vi "Draw TextBox.vi"(7 "heading (rad)":dbl, 9 "draw options":T1={"Outer Border Color"=0, "Inner Border Color"=6316128, "Outer Gradient Color"=2565927, "Inner Gradient Color"=16860, "Compass North Pointer Color"=16711680, "Compass Pointer Color 1"=13355429, "Compass Pointer Color 2"=14934973, "Direction Pointer Color"=16765184, "Text Box Outline Color"=13355429, "Text Box Background Color"=14934973, "Scale Color"=16448250, "Text Color"=0, "Draw Gradient"=TRUE, "Draw Rose"=TRUE, "Simple Scale"=TRUE, "Draw Text"=FALSE, "Font Name"="Helvetica", "Angle Units"=enum."Degrees"}, 10 "draw area cache":T3, 11 "picture in":picture) -> (3 "picture out":picture)   [LabVIEW 2017, in "NI_Robotics_Compass Picture.lvlib"]
uses:
  <vilib>/robotics/Controls/Compass Indicator/Compass Picture/NI_Robotics_Compass Picture.lvlib
  <vilib>/robotics/Controls/Compass Indicator/Compass Picture/Draw Area State.ctl
  <vilib>/Utility/miscctls.llb/LVBoundsTypeDef.ctl
  <vilib>/robotics/Controls/Compass Indicator/Compass Picture/Draw Options.ctl
  <vilib>/robotics/Controls/Utilities/Angle Units.ctl
  <vilib>/picture/picture.llb/Get Text Rect.vi
  <vilib>/Utility/AngleManip/Radians to Degrees.vi
  <vilib>/Utility/AngleManip/Radians to Degrees (Scalar DBL).vi
  <vilib>/robotics/Controls/Utilities/NI_Robotics_Control Utilities.lvlib
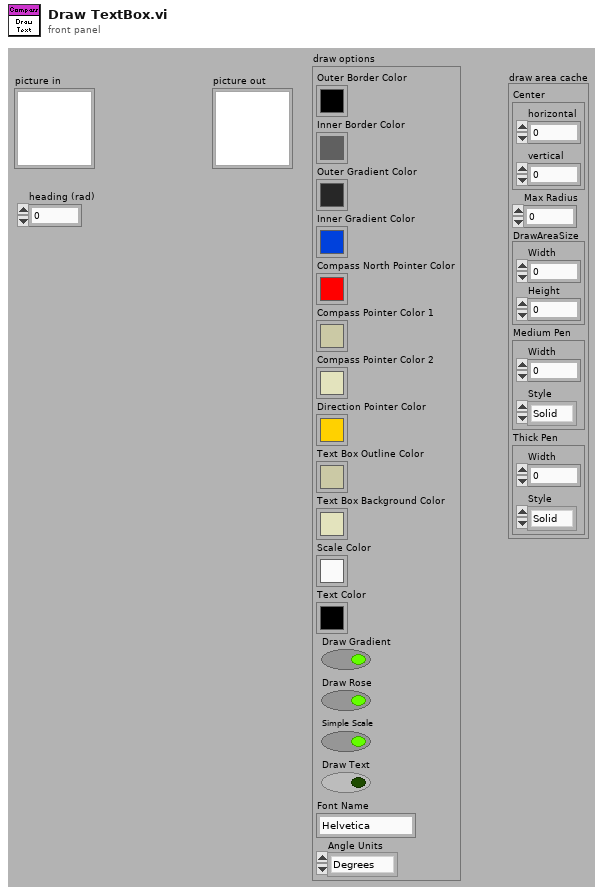
[diagram p1: front panel]
types:
  T1 = typedef "NI_Robotics_Compass Picture.lvlib/Draw Options.ctl" = cluster{"Outer Border Color":u32, "Inner Border Color":u32, "Outer Gradient Color":u32, "Inner Gradient Color":u32, "Compass North Pointer Color":u32, "Compass Pointer Color 1":u32, "Compass Pointer Color 2":u32, "Direction Pointer Color":u32, "Text Box Outline Color":u32, "Text Box Background Color":u32, "Scale Color":u32, "Text Color":u32, "Draw Gradient":bool, "Draw Rose":bool, "Simple Scale":bool, "Draw Text":bool, "Font Name":string, "Angle Units":T2}
  T2 = typedef "NI_Robotics_Control Utilities.lvlib/Angle Units.ctl" = enum16{"Radians", "Degrees"}
  T3 = typedef "NI_Robotics_Compass Picture.lvlib/Draw Area State.ctl" = cluster{"Center":cluster{"horizontal":i16, "vertical":i16}, "Max Radius":dbl, "DrawAreaSize":T4, "Medium Pen":cluster{"Width":u16, "Style":enum32{"Solid", "Dash", "Dot", "DashDot", "DashDotDot"}}, "Thick Pen":cluster{"Width":u16, "Style":enum32{"Solid", "Dash", "Dot", "DashDot", "DashDotDot"}}}
  T4 = typedef "LVBoundsTypeDef.ctl" = cluster{"Width":u32, "Height":u32}
  T5 = cluster{"horizontal":enum16{"left", "center", "right"}, "vertical":enum16{"top", "center", "bottom"}}
  T6 = enum16{"User-specified Font", "Application Font", "System Font", "Dialog Font"}
  T7 = cluster{"Width":u16, "Style":enum32{"Solid", "Dash", "Dot", "DashDot", "DashDotDot"}}
  T8 = cluster{"left":i16, "top":i16, "right":i16, "bottom":i16}
  T9 = cluster{"Font Name:":string, "Size":i16, "Strikeout?":bool, "Italic?":bool, "Underline?":bool, "Outline?":bool, "Shadow?":bool, "Bold?":bool}
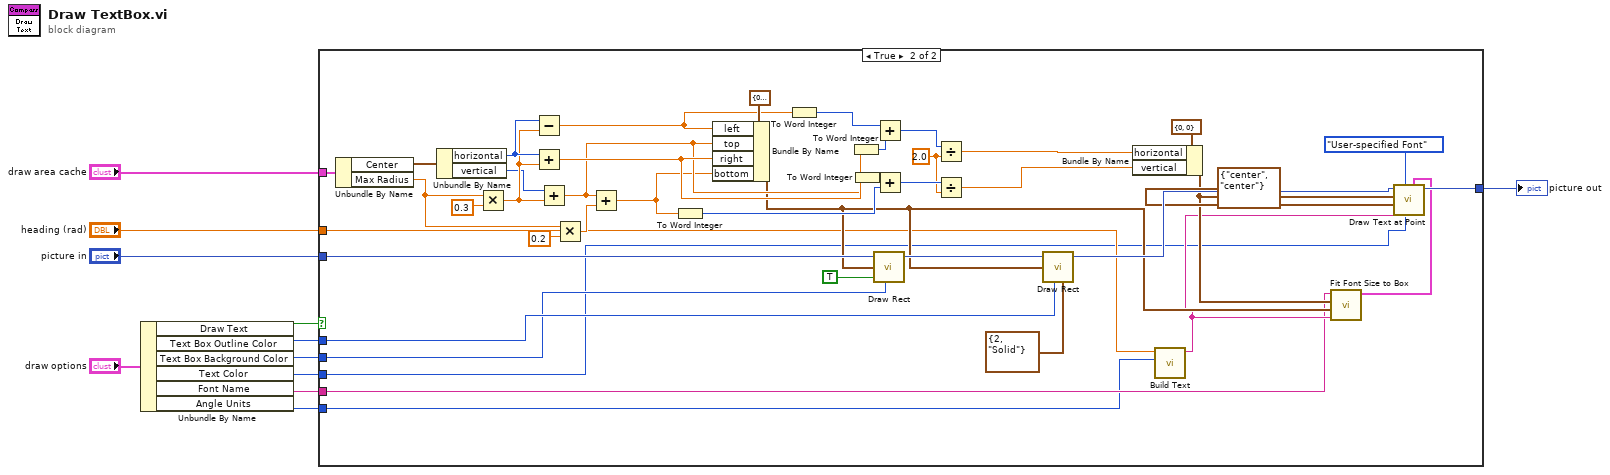
[diagram p0: block diagram]
diagram:
  n1 = Unbundle By Name("draw options") -> ("Draw Text"=w1:bool, "Text Box Outline Color"=w6:u32, "Text Box Background Color"=w5:u32, "Text Color"=w4:u32, "Font Name"=w3:string, "Angle Units"=w2:T2)
  n2 = case shown="True" w1 {
    tunnel: [w12 w54] -> w11
    tunnel: "picture in" -> [w12 w42]
    tunnel: "draw area cache" -> [_ w33]
    tunnel: "heading (rad)" -> [_ w19]
    tunnel: w6 -> [_ w17]
    tunnel: w5 -> [_ w16]
    tunnel: w4 -> [_ w15]
    tunnel: w3 -> [_ w14]
    tunnel: w2 -> [_ w13]
    frame False {
    }
    frame True {
      w39 = 2.0 ("y")
      n3 = Unbundle By Name(w33) -> ("Center"=w32:cluster{"horizontal":i16, "vertical":i16}, "Max Radius"=w31:dbl)
      n4 = Unbundle By Name(w32) -> ("horizontal"=w49:i16, "vertical"=w44:i16)
      n5 = Multiply(x=w31, y=0.3) -> (x*y=w46:dbl)
      n6 = Subtract(x=w49, y=w46) -> (x-y=w30:dbl)
      n7 = Add(x=w49, y=w46) -> (x+y=w29:dbl)
      n8 = Add(x=w44, y=w46) -> (x+y=w28:dbl)
      n9 = Multiply(x=w31, y=0.2) -> (x*y=w48:dbl)
      n10 = Add(x=w28, y=w48) -> (x+y=w27:dbl)
      n11 = To Word Integer(number=w27) -> (16bit integer=w23:i16)
      n12 = Bundle By Name(cluster=T8 {"left"=0, "top"=0, "right"=0, "bottom"=0} ("rect"), "left"=w30, "top"=w28, "right"=w29, "bottom"=w27) -> (w21:T8)
      n13 = To Word Integer(number=w30) -> (16bit integer=w26:i16)
      n14 = To Word Integer(number=w29) -> (16bit integer=w24:i16)
      n15 = To Word Integer(number=w28) -> (16bit integer=w25:i16)
      n16 = call <vilib>:"Draw Rect.vi"("picture"=w42, "rect"=w21, "fill?(F)"=TRUE, "color(black)"=w16) -> ("new picture"=w50:picture)  [unwired: 5 in]
      n17 = Add(x=w26, y=w24) -> (x+y=w41:i16)
      n18 = Add(x=w25, y=w23) -> (x+y=w40:i16)
      n19 = Divide(x=w41, y=w39) -> (x/y=w37:dbl)
      n20 = Divide(x=w40, y=w39) -> (x/y=w36:dbl)
      n21 = call <vilib>:"Draw Rect.vi"("picture"=w50, "rect"=w21, "color(black)"=w17, "pen"=T7 {"Width"=2, "Style"=enum."Solid"}) -> ("new picture"=w53:picture)  [unwired: 5 in]
      n22 = Bundle By Name(cluster=cluster{"horizontal":i16, "vertical":i16} {"horizontal"=0, "vertical"=0} ("origin(0,0)"), "horizontal"=w37, "vertical"=w36) -> (w22:cluster{"horizontal":i16, "vertical":i16})
      n23 = call <vilib>:"Build Text.vi"("angle units"=w13, "heading (rad)"=w19) -> ("text"=w18:string)  [unwired: 9 in]
      n24 = call <vilib>:"Fit Font Size to Box.vi"("text"=w18, "box rect"=w21, "box center"=w22, "font name"=w14) -> ("font"=w20:T9)  [unwired: 7 in]
      n25 = call <vilib>:"Draw Text at Point.vi"("[user-specified font]"=w20, "text color(black)"=w15, "desired font(Application)"=T6."User-specified Font", "text"=w18, "alignment(left, top)"=T5 {"horizontal"=enum."center", "vertical"=enum."center"}, "origin"=w22, "picture"=w53) -> ("new picture"=w54:picture)  [unwired: 3 in, 1 out]
    }
  }
  "picture out" <- w11
